vi "WPI_AnalogOutputSetVoltage.vi"(8 "error in (no error)":errorcluster, 10 "Voltage":dbl min=0.0 max=5.0, 11 "AODeviceRef":T1={"DevStatus"={"status"=FALSE, "code"=0, "source"=""}, "AO Channel"=enum."Invalid"}) -> (0 "error out":errorcluster, 3 "AODeviceRef":T1={"DevStatus"={"status"=FALSE, "code"=0, "source"=""}, "AO Channel"=enum."Invalid"})   [LabVIEW 2017]
doc: "Sets the voltage on the analog output channel. The output range is 0 to 5V.\n\nThis software is licensed. Open the labview\\readme\\WPI Robotics Library Open Source License.txt file for more information."
uses:
  <vilib>/Rock Robotics/WPI/AnalogOutput/WPI_AOChannelDevRef.ctl
  <vilib>/Rock Robotics/WPI/AnalogOutput/WPI_AnalogOutputChannel.ctl
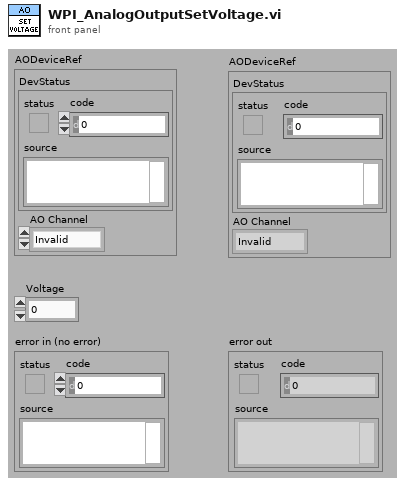
[diagram p1: front panel]
types:
  T1 = typedef "WPI_AOChannelDevRef.ctl" = cluster{"DevStatus":errorcluster, "AO Channel":T2}
  T2 = typedef "WPI_AnalogOutputChannel.ctl" = enum8{"AO MXP 0", "AO MXP 1", "Invalid"}
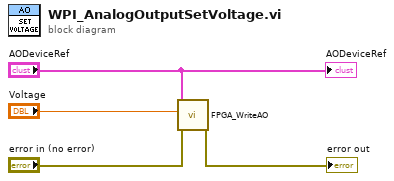
[diagram p0: block diagram]
diagram:
  n1 = call <vilib>:"FPGA_WriteAO.vi"("error in"="error in (no error)", "Voltage"="Voltage", "AO Reference"="AODeviceRef") -> ("error out"=→"error out":errorcluster)  [unwired: 7 in, 1 out]
  "AODeviceRef" <- "AODeviceRef"
